vi "Generate SysDef Path.vi"(3 "reference in":refnum<class "FPGA Addon DMA Waveform Status Channel System Tests.lvclass">=refnum) -> (0 "SysDef path":path, 1 "reference out":refnum<class "FPGA Addon DMA Waveform Status Channel System Tests.lvclass">)   [LabVIEW 2019, in "FPGA Addon DMA Waveform Status Channel System Tests.lvclass"]
uses:
  FPGA Addon DMA Waveform Status Channel System Tests.lvclass
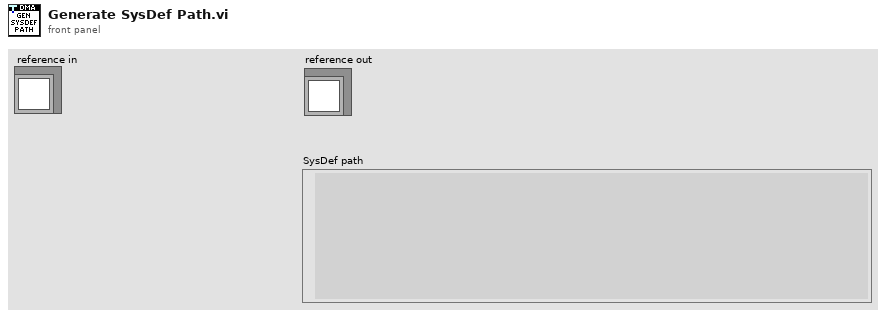
[diagram p1: front panel]
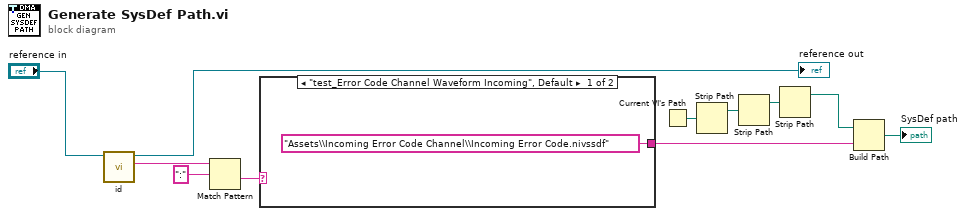
[diagram p0: block diagram]
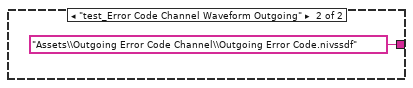
[diagram p2: hidden frame]
diagram:
  n1 = call-dynamic "id.vi"("TestCase in"="reference in") -> ("id"=w10:string, "TestCase out"=→"reference out":refnum<class "FPGA Addon DMA Waveform Status Channel System Tests.lvclass">)  [unwired: 7 in, 2 out]
  n2 = Match Pattern(string=w10, regular expression=":") -> (after substring=w8:string)  [unwired: 1 in, 3 out]
  n3 = case shown="\"test_Error Code Channel Waveform Incoming\", Default" w8 {
    tunnel: ["Assets\\Incoming Error Code Channel\\Incoming Error Code.nivssdf" ("name or relative path") "Assets\\Outgoing Error Code Channel\\Outgoing Error Code.nivssdf" ("name or relative path")] -> w3
    frame "test_Error Code Channel Waveform Incoming", Default {
    }
    frame "test_Error Code Channel Waveform Outgoing" {
    }
  }
  n4 = Current VI's Path() -> (path=w6:path)
  n5 = Strip Path(path=w6) -> (stripped path=w5:path)  [unwired: 1 out]
  n6 = Strip Path(path=w5) -> (stripped path=w4:path)  [unwired: 1 out]
  n7 = Strip Path(path=w4) -> (stripped path=w2:path)  [unwired: 1 out]
  n8 = Build Path(base path=w2, name or relative path=w3) -> (appended path=→"SysDef path":path)
